vi "Lvi Subsystem Set Quad Encoder.vi"(7 "X4Scaling":bool, 8 "error in (no error)":errorcluster, 9 "IndexMode":i32, 10 "ClockPrescale":u32, 11 "TaskRef":i32) -> (0 "error out":errorcluster, 2 "function return":i32, 3 "TaskRef out":i32)   [LabVIEW 2016, in "DtLvLink.lvlib"]
doc: "Calls directly into the entry points of the DLL of the Data Acq SDK to create one or more virtual channels, add them to a task, and configure the task with the specified settings to determine the current position, in counts, of a quadrature encoder input. This VI is used by the higher-level VI, DtOLCreateTask."
uses:
  <userlib>/LV-Link3/DtLvLink.lvlib
  <userlib>/LV-Link3/DtLvLink_32.dll
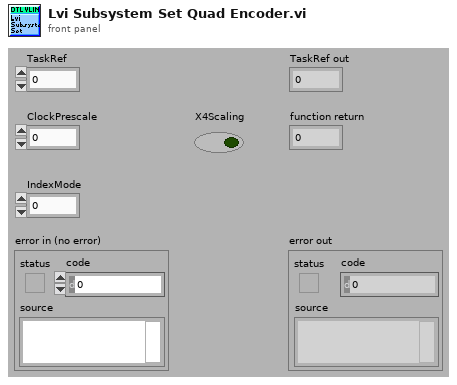
[diagram p1: front panel]
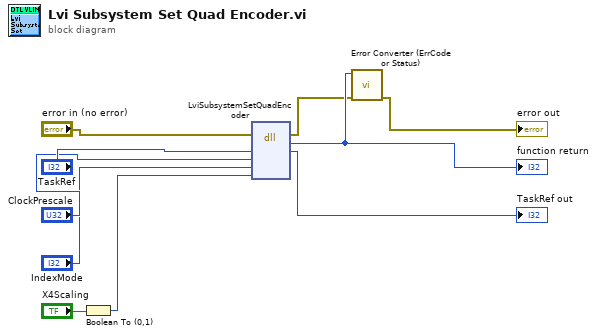
[diagram p0: block diagram]
diagram:
  n1 = Boolean To (0,1)(Boolean="X4Scaling") -> (0, 1=w4:i16)
  n2 = dll-call lib="C:/Program Files (x86)/National Instruments/LabVIEW 2016/user.lib/LV-Link3/DtLvLink_32.*" fn="LviSubsystemSetQuadEncoder"(error in="error in (no error)", "TaskRef"="TaskRef", "ClockPrescale"="ClockPrescale", "IndexMode"="IndexMode", "X4Scaling"=w4) -> (error out=w2:errorcluster, w10:i32, "TaskRef"=→"TaskRef out":i32)  [unwired: 5 in, 1 out]
  "function return" <- w10
  n3 = call <userlib>:"Error Converter (ErrCode or Status).vi"("error in (no error)"=w2, "error code"=w10) -> ("error out"=→"error out":errorcluster)  [unwired: 9 in]
